vi "Network Command Engine.vi"(8 "error in (no error)":errorcluster, 11 "State Variables":T1) -> (0 "error out":errorcluster)   [LabVIEW 2015, in "Instrument Addon Engine.lvlib"]
uses:
  Instrument Addon Engine.lvlib
  Types/Engine State Variables.ctl
  <vilib>/NI/NI VeriStand Inline Async API/_VS Inline Async API/Process/Process.lvclass
  Types/TCP Refs.ctl
  <vilib>/NI/STM/Connection Manager/TCP/Advanced/TCP Connection Manager Reference.ctl
  <vilib>/NI/STM/Connection Manager/TCP/Advanced/TCP Connection Manager State Variables.ctl
  <vilib>/NI/STM/TCP/TCP Connection Info.ctl
  <vilib>/NI/STM/SubVIs/MetaDataElement.ctl
  <vilib>/NI/STM/Connection Manager/TCP/TCP Connection Properties.ctl
  <vilib>/NI/AMC/Message Queue.ctl
  <vilib>/NI/AMC/Message.ctl
  <vilib>/NI/Tools/Keyed Array/KeyedArray.ctl
  <vilib>/NI/NI VeriStand Inline Async API/_Data Access Engine/Access Type Classes/Write/Write.lvclass
  <vilib>/NI/NI VeriStand Inline Async API/_Data Access Engine/Access Type Classes/Read/Read.lvclass
  <vilib>/NI/NI VeriStand Inline Async API/_Data Access Engine/Access Type Classes/ReadWrite/ReadWrite.lvclass
  <vilib>/NI/STM/Connection Manager/TCP/TCP Connection Method.ctl
  <vilib>/NI/STM/TCP/TCP Read Options.ctl
  <vilib>/NI/NI VeriStand Inline Async API/_VS Inline Async API/Process/Process.lvclass/Process.ctl
  <vilib>/NI/STM/TCP/Get Connection Reference (TCP).vi
  <vilib>/NI/AMC/Create Single Message.vi
  <vilib>/NI/AMC/Update Message Routing Info.vi
  <vilib>/NI/Tools/Keyed Array/Map String.vi
  <vilib>/NI/AMC/Read Termination Message.vi
  <vilib>/NI/NI VeriStand Inline Async API/_VS Inline Async API/Error Handling Process/SubVIs/Error.ConvertArray.vi
  <vilib>/NI/Tools/String/Get Case Matching.vi
  <vilib>/NI/STM/TCP/Write Message (TCP).vi
  <vilib>/NI/AMC/Globals.vi
  <vilib>/NI/AMC/Send Message.vi
  Shared/Constants.vi
  <vilib>/NI/STM/TCP/Read Message (TCP).vi
  <vilib>/NI/AMC/AMC.lvlib
  <vilib>/NI/Tools/Keyed Array/Tools_KeyedArray.lvlib
  Shared/Instrument Addon Shared.lvlib
  <vilib>/NI/STM/NI STM.lvlib
  <vilib>/NI Veristand/Custom Device Tools/Custom Device Utility Library/Custom Device Utility Library.lvlib
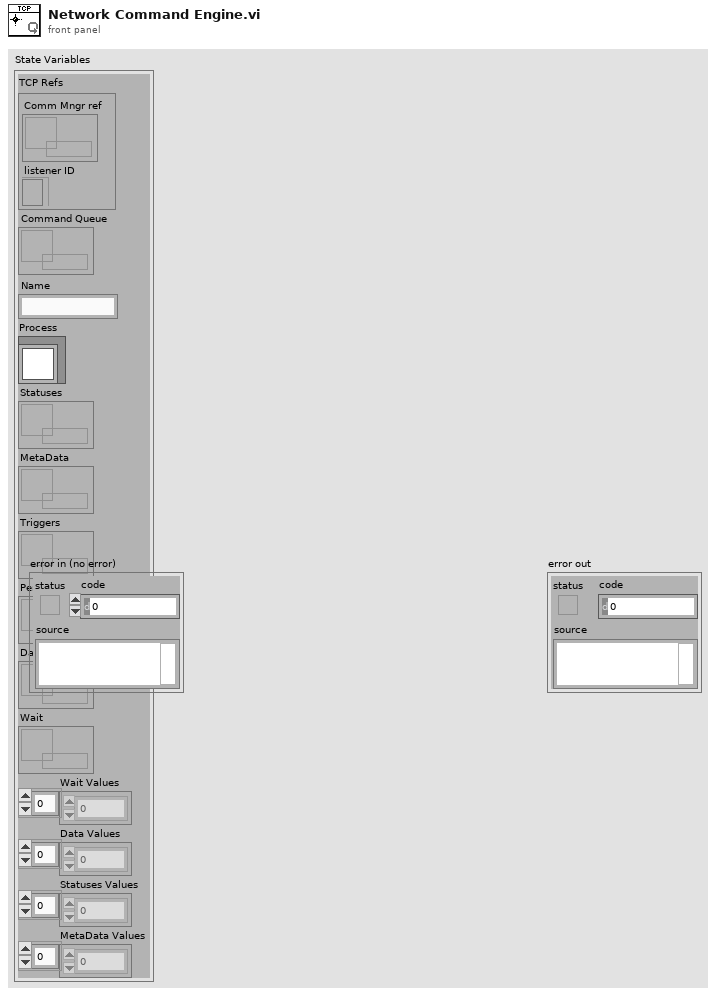
[diagram p1: front panel]
types:
  T1 = typedef "Instrument Addon Engine.lvlib/Engine State Variables.ctl" = cluster{"TCP Refs":T2, "Command Queue":T4, "Name":string, "Process":refnum<class "Process.lvclass">, "Statuses":refnum<data-value>, "MetaData":refnum<data-value>, "Triggers":refnum<data-value>, "Periodic Enable":refnum<data-value>, "Data":refnum<data-value>, "Wait":refnum<data-value>, "Wait Values":dbl[], "Data Values":dbl[], "Statuses Values":dbl[], "MetaData Values":dbl[]}
  T2 = typedef "Instrument Addon Engine.lvlib/TCP Refs.ctl" = cluster{"Comm Mngr ref":T3, "listener ID":refnum<k5>}
  T3 = typedef "TCP Connection Manager Reference.ctl" = refnum<data-value>
  T4 = typedef "AMC.lvlib/Message Queue.ctl" = refnum<queue>
  T5 = typedef "NI STM.lvlib/TCP Connection Method.ctl" = enum16{"Initialize", "Add Connection", "Set Properties", "Get Connection(s)", "Remove Connection", "Remove All Connections", "Get Connection Count"}
  T6 = typedef "NI STM.lvlib/TCP Connection Info.ctl" = cluster{"connection ID":refnum<k5>, "meta data":T7[]}
  T7 = typedef "NI STM.lvlib/MetaDataElement.ctl" = string
  T8 = typedef "NI STM.lvlib/TCP Read Options.ctl" = cluster{"ignore timeout error":bool, "timeout ms (1000)":i32}
  T9 = typedef "Tools_KeyedArray.lvlib/KeyedArray.ctl" = cluster{"keys":string[], "values":string[]}
  T10 = typedef "NI STM.lvlib/TCP Connection Properties.ctl" = cluster{"Name":string, "Address":string, "Custom":string}
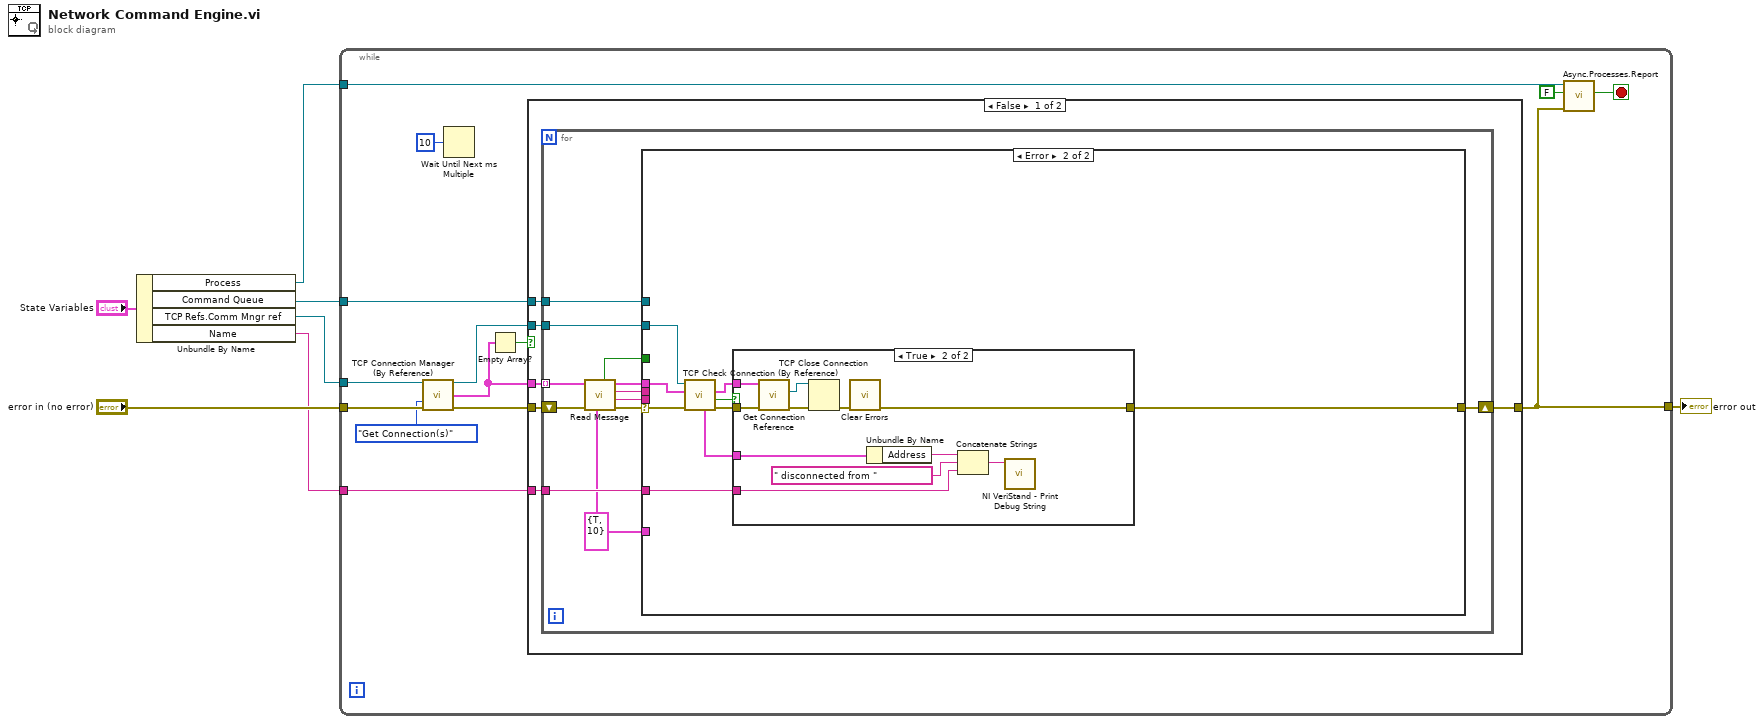
[diagram p0: block diagram]
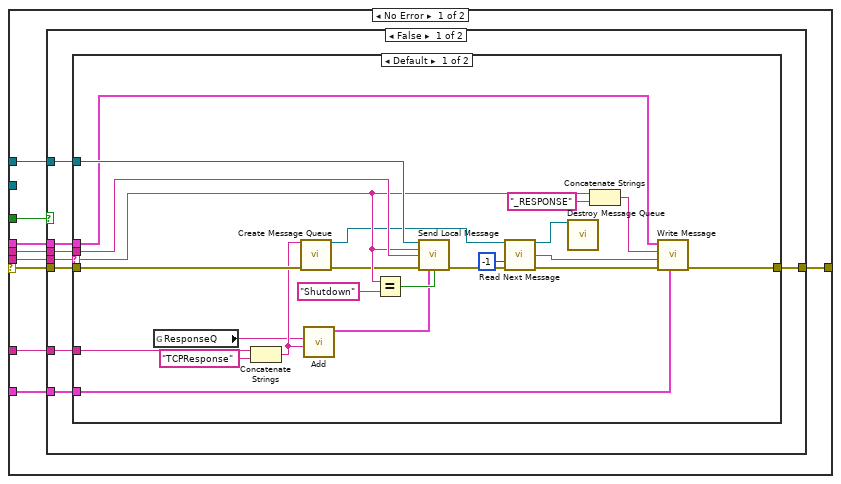
[diagram p2: hidden frame]
diagram:
  n1 = Unbundle By Name("State Variables") -> ("Process"=w7:refnum<class "Process.lvclass">, "Command Queue"=w1:T4, "TCP Refs.Comm Mngr ref"=w5:T3, "Name"=w2:string)
  n2 = while {
    tunnel: "error in (no error)" -> [w18]
    tunnel: [w9] -> w3
    tunnel: w5 -> [w14]
    tunnel: w7 -> [w13]
    tunnel: w2 -> [w12]
    tunnel: w1 -> [w10]
    stop <- w15 stop-if-true
    n3 = call <vilib>:"TCP Connection Manager (By Reference).vi"("connection manager ref in"=w14, "method"=TCP_Connection_Method."Get Connection(s)", "error in"=w18) -> ("connection manager ref out"=w16:T3, "all connections"=w19:T6[], "error out"=w17:errorcluster)  [unwired: 6 in, 4 out]
    n4 = Wait Until Next ms Multiple(millisecond multiple=u32 10 ("STM Update Rate")) -> ()  [unwired: 1 out]
    n5 = Empty Array?(array=w19) -> (empty?=w20:bool)
    n6 = case shown="False" w20 {
      tunnel: w19 -> [w27 _]
      tunnel: w17 -> [w23 w103]
      tunnel: w16 -> [w26 _]
      tunnel: [w25 w103] -> w9
      tunnel: w12 -> [w24 _]
      tunnel: w10 -> [w22 _]
      frame False {
        n7 = for {
          tunnel: w27 -> [w34] mode=indexing
          tunnel: w26 -> [w39]
          shift-right: [w38] -> w25
          shift-left: w23 -> [w36]
          tunnel: w24 -> [w37]
          tunnel: w22 -> [w29]
          w28 = T8 {"ignore timeout error"=TRUE, "timeout ms (1000)"=10} ("options")
          n8 = call-poly <vilib>:"Read Message.vi"("options"=w28, "error in"=w36, "connection info in"=w34) -> ("error out"=w35:errorcluster, "name"=w31:T7, "data string"=w32:string, "connection info out"=w33:T6, "timed out?"=w30:bool)  [unwired: 3 in, 1 out]
          n9 = case shown="Error" w35 {
            selector: w35 -> [w48 w85]
            tunnel: w39 -> [_ w87]
            tunnel: w33 -> [w42 w86]
            tunnel: [w47 w84] -> w38
            tunnel: w37 -> [w41 w83]
            tunnel: w32 -> [w46 _]
            tunnel: w31 -> [w45 _]
            tunnel: w30 -> [w44 _]
            tunnel: w29 -> [w43 _]
            tunnel: w28 -> [w40 _]
            frame No Error {
              n10 = case shown="False" w44 {
                tunnel: w48 -> [w53 w81]
                tunnel: [w56 w81] -> w47
                tunnel: w46 -> [w51 _]
                tunnel: w45 -> [w52 _]
                tunnel: w43 -> [w55 _]
                tunnel: w42 -> [w54 _]
                tunnel: w41 -> [w50 _]
                tunnel: w40 -> [w49 _]
                frame False {
                  n11 = case shown="Default" w52 {
                    selector: w52 -> [w70 _]
                    tunnel: w53 -> [w79 w80]
                    tunnel: [w74 w80] -> w56
                    tunnel: w51 -> [w78 _]
                    tunnel: w55 -> [w76 _]
                    tunnel: w54 -> [w73 _]
                    tunnel: w50 -> [w77 _]
                    tunnel: w49 -> [w68 _]
                    frame Default {
                      n12 = global read "Constants.vi" "ResponseQ"() -> (w57:string)
                      n13 = Concatenate Strings(w77, "TCPResponse" ("message name")) -> (w62:string)
                      n14 = call <vilib>:"Create Message Queue.vi"("message queue name"=w62, "error in"=w79) -> ("message queue out"=w60:T4, "error out"=w65:errorcluster)  [unwired: 12 in]
                      n15 = call <vilib>:"Add.vi"("value"=w62, "key"=w57) -> ("array out"=w63:T9)  [unwired: 3 in, 2 out]
                      n16 = Equal?(x=w70, y="Shutdown" ("x")) -> (x = y?=w67:bool)
                      n17 = call <vilib>:"Send Local Message.vi"("message queue in"=w76, "message name"=w70, "message value"=w78, "error in"=w65, "message attributes"=w63, "priority message (F)"=w67) -> ("error out"=w61:errorcluster)  [unwired: 7 in, 2 out]
                      n18 = call <vilib>:"Read Next Message.vi"("message queue in"=w60, "timeout (1 ms)"=-1, "error in"=w61) -> ("message queue out"=w58:T4, "message value"=w72:string, "error out"=w75:errorcluster)  [unwired: 5 in, 5 out]
                      n19 = call <vilib>:"Destroy Message Queue.vi"("message queue in"=w58) -> ()  [unwired: 12 in, 3 out]
                      n20 = Concatenate Strings(w70, "_RESPONSE" ("string")) -> (w69:string)
                      n21 = call-poly <vilib>:"Write Message.vi"("options"=w68, "error in"=w75, "data"=w72, "name"=w69, "connection info in"=w73) -> ("error out"=w74:errorcluster)  [unwired: 5 in, 1 out]
                    }
                    frame "" {
                    }
                  }
                }
                frame True {
                }
              }
            }
            frame Error {
              n22 = call <vilib>:"TCP Check Connection (By Reference).vi"("error in"=w85, "connection in"=w86, "connection manager ref in"=w87) -> ("error out"=w90:errorcluster, "disconnected?"=w88:bool, "connection out"=w89:T6, "properties out"=w82:T10)  [unwired: 4 in, 1 out]
              n23 = case shown="True" w88 {
                tunnel: [w91 w99] -> w84
                tunnel: w90 -> [w91 w102]
                tunnel: w89 -> [_ w97]
                tunnel: w83 -> [_ w93]
                tunnel: w82 -> [_ w92]
                frame False {
                }
                frame True {
                  n24 = call-poly <vilib>:"Get Connection Reference.vi"("error in"=w102, "connection info in"=w97) -> ("error out"=w101:errorcluster, "connection ID out"=w100:refnum<k5>)  [unwired: 7 in, 1 out]
                  n25 = TCP Close Connection(connection ID=w100, error in (no error)=w101) -> (error out=w98:errorcluster)  [unwired: 1 in, 1 out]
                  n26 = call <vilib>:"Clear Errors.vi"("error in (no error)"=w98) -> ("error out"=w99:errorcluster)  [unwired: 5 in, 1 out]
                  n27 = Unbundle By Name(w92) -> ("Address"=w94:string)
                  n28 = Concatenate Strings(w94, " disconnected from " ("string"), w93) -> (w96:string)
                  n29 = call <vilib>:"NI VeriStand - Print Debug String.vi"("Message"=w96) -> ()  [unwired: 10 in, 1 out]
                }
              }
            }
          }
        }
      }
      frame True {
      }
    }
    n30 = call <vilib>:"Async.Processes.Report.vi"("Error"=w9, "Stop on Error?"=FALSE, "Process in"=w13) -> ("Stop"=w15:bool)  [unwired: 7 in, 1 out]
  }
  "error out" <- w3
